vi "ReversedEngineering StateQueuedSettings.vi"(5 "error in (no error)":errorcluster) -> (15 "Cancelled":bool, 19 "error out":errorcluster)   [LabVIEW 2012]
uses:
  <resource>/Framework/Providers/Open_GDS/UML/UMLEditor/UMLEditor_StoredPathes.ctl
  <resource>/Framework/Providers/Open_GDS/UML/ContextHelp/ContextHelp_HelpTexts.ctl
  <resource>/Framework/Providers/Open_GDS/ClassProviders/Common/File/File_StoredPathesActions.ctl
panel:
  in  "Help":bool
  in  "VI-Name":string caption="VI-Name that inserts an array of states-transitions\nin the queued state machine."
  in  "Cancel Button":bool
  in  "OK Button":bool
  in  "Path":path
  # "E.g."
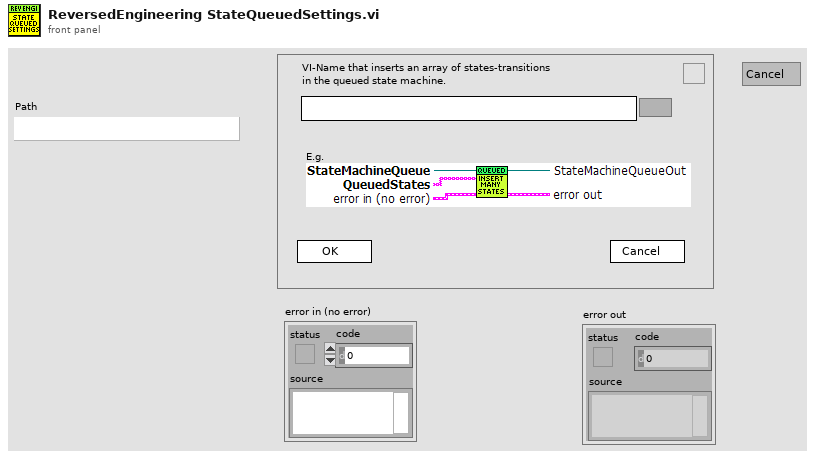
[diagram p1: front panel]
types:
  T1 = typedef "UMLEditor_StoredPathes.ctl" = enum16{"LastSearchPath", "QueuedArrayStateVI", "ClassBasePath", "ViTemplatePath", "ApplicationTemplatePath", "IniFilePath", "WizDir", "RevPlugInPath"}
  T2 = typedef "ContextHelp_HelpTexts.ctl" = enum16{"None(Hide)", "Default", "Help", "Welcome", "GettingStarted", "ClassDiagram_Help", "SequenceDiagram_Help", "UseCaseDiagram_Help", "BSelect", "BClass", "BInterface", "BPackage", "BNote", "BDependency", "BInheritance", "BInterfaceImplementation", "BAssociation", "BAggregation", "BCompAggregation", "BNoteConnector", "BObject", "BActionBar", "BCall", "BSystem", "BActor", "BUseCase", "BGeneralization", "BIncludes", "BExtends", "BUseCaseDiagramAssociation", "ClassRelationshipEdge editDialog_Bent Style", "ClassRelationshipEdge editDialog_RelationType", "ClassRelationshipEdge editDialog_Reverse association", "ClassRelationshipEdge editDialog_Start label", "ClassRelationshipEdge editDialog_Middle label", "ClassRelationshipEdge editDialog_End label", "UMLEditor reversedEngineering_Pathes", "ReversedEngineering StateReverseDialog_Help", "ReversedEngineering StateQueuedSettings_Help", "UMLEditor reversedEngineering_AddTopVIs", "UMLEditor reversedEngineering_AddClasses", "UMLEditor reversedEngineering_AddDirs", "UMLEditor reversedEngineering_Recursively", "UMLEditor reversedEngineering_Remove", "UMLEditor reversedEngineering_ClearList", "UMLEditor reversedEngineering_HideSubAss", "UMLEditor reversedEngineering_CreateTypes", "UMLEditor reversedEngineering_OnlyInheritance", "UMLEditor reversedEngineering_CreateApplication", "UMLEditor reversedEngineering_OK", "UMLEditor reversedEngineering_Cancel", "UMLEditor reversedEngineering_Help", "UMLEditor createWizardScriptFile_ScriptfilePath", "UMLEditor createWizardScriptFile_ClassPath", "UMLEditor createWizardScriptFile_Use", "UMLEditor createWizardScriptFile_PrivateDirName", "UMLEditor createWizardScriptFile_DirAppend", "UMLEditor createWizardScriptFile_Separator Character", "UMLEditor createWizardScriptFile_OK", "UMLEditor createWizardScriptFile_Cancel", "UMLEditor createWizardScriptFile_Help", "ClassNode editDialog_Class Name", "InterfaceNode editDialog_Class Name", "ClassNode editDialog_Attribute", "ClassNode editDialog_Methods", "InterfaceNode editDialog_Methods", "ClassNode editDialog_connection", "InterfaceNode editDialog_connection", "ClassNode editDialog_StereoType", "ClassNode editDialog_ShowAttrib", "ClassNode editDialog_ShowMethods", "ClassNode editDialog_ClassPath", "ClassNode editDialog_AddAttribute", "ClassNode editDialog_AddMethod", "InterfaceNode editDialog_AddMethod", "ClassNode AttributeGuide_AttributeName", "ClassNode AttributeGuide_Array?", "ClassNode AttributeGuide_Data Type", "ClassNode AttributeGuide_RefName", "ClassNode AttributeGuide_Preview", "ClassNode AttributeGuide_OK", "ClassNode AttributeGuide_Cancel", "ClassNode MethodGuide_Visibility", "ClassNode MethodGuide_Method Name", "ClassNode MethodGuide_Preview", "ClassNode MethodGuide_OK", "ClassNode MethodGuide_Cancel", "CallNode EditCallProperties_AllButtons", "ObjectNode EditObjectlProperties_AllButtons", "ActorNode EditActorProperties_AllButtons", "UseCaseRelationshipNode EditUseCaselProperties_AllButtons", "UseCaseNode EditUseCaselProperties_AllButtons", "SystemNode EditSystemProperties_AllButtons", "ReversedEngineering UpdateAttributes_AllButtons", "StateNode editDialog_AllButtons", "StateTransition editDialog_AllButtons", "ArrangeNodes Main_Picture", "ArrangeNodes Main_Zoom", "ArrangeNodes Main_Auto Zoom", "ArrangeNodes Main_shorten", "ArrangeNodes Main_Min Length", "ArrangeNodes Main_Max Length", "ArrangeNodes Main_increase", "ArrangeNodes Main_decrease", "ArrangeNodes Main_Shake", "ArrangeNodes Main", "BState", "BInitialState", "BFinalState", "BStateTransition", "StateDiagram_Help", "StateDiagram_PropertiesAllButtons", "ReversedEngineering StateReverseDialog_ClearStates", "ReversedEngineering StateReverseDialog_UseQueuedStateMachines", "ReversedEngineering StateReverseDialog_QueuedSettings", "ReversedEngineering StateReverseDialog_SearchForVIs", "ReversedEngineering StateReverseDialog_SearchCriteria", "OptionsDialog_ClassBasePath", "OptionsDialog_VIPath", "OptionsDialog_ApplicationPath", "OptionsDialog_WizDir", "OptionsDialog_IniFilePath", "OptionsDialog_DefineColors", "OptionsDialog_Help", "OptionsDialog_CreateTypes", "ClassRelationshipEdge editDialog_SplitWire"}
  T3 = typedef "ContextHelp_ShowType.ctl" = cluster{"Header":string, "Picture":picture, "Text":string}
  T4 = typedef "File_StoredPathesActions.ctl" = enum16{"Get Path", "Set Path", "Delete Path", "Clear All Paths"}
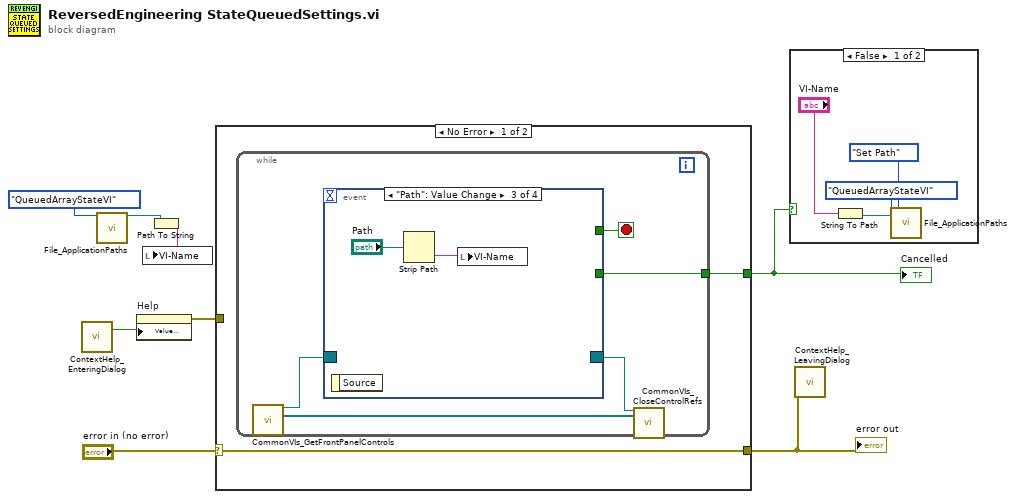
[diagram p0: block diagram]
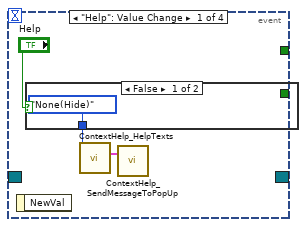
[diagram p3: hidden frame]
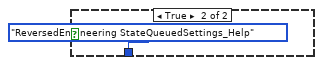
[diagram p4: hidden frame]
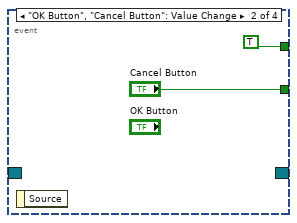
[diagram p5: hidden frame]
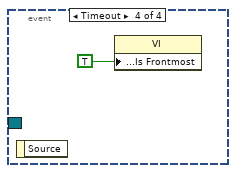
[diagram p6: hidden frame]
diagram:
  n1 = call <resource>:"ContextHelp_EnteringDialog.vi"() -> ("HelpStatus"=w7:bool)  [unwired: 1 in, 18 out]
  n2 = call <resource>:"File_ApplicationPaths.vi"("PathName"=UMLEditor_StoredPathes."QueuedArrayStateVI" ("UMLPathes")) -> ("Path Out"=w2:path)  [unwired: 3 in, 15 out]
  n3 = property on="Help" class="Bool (strict)"("Value (Signaling)"=w7) -> (error out=w6:errorcluster)  [unwired: 2 in, 1 out]
  n4 = Path To String(path=w2) -> (string=w1:string)
  n5 = local write "VI-Name"(w1) -> ()
  n6 = case shown="No Error" "error in (no error)" {
    selector: "error in (no error)" -> [w10 w26]
    tunnel: [w10 w26] -> w5
    tunnel: w6 -> [_ _]
    tunnel: [w9 _] -> w4
    frame No Error {
      n7 = while {
        tunnel: [w11] -> w9
        stop <- w12 stop-if-true
        n8 = call <resource>:"CommonVIs_GetFrontPanelControls.vi"() -> ("Event Registration Refnum"=w14:refnum<event-registration>, "ControlRefs"=w15:refnum<vi>[])  [unwired: 2 in, 16 out]
        n9 = event shown="[2] \"Path\": Value Change" {
          selector: w14 -> [_ _ _ _]
          dyn-events: [_ _ _ _] -> w13
          timeout: _ -> [_ _ _ _]
          tunnel: [_ TRUE _ _] -> w12
          tunnel: [_ "Cancel Button" _ _] -> w11
          event "Help": Value Change {
            n10 = event-data() -> ()  [unwired: 2 out]
            n11 = case shown="False" "Help" {
              tunnel: [ContextHelp_HelpTexts."None(Hide)" ("HelpText") ContextHelp_HelpTexts."ReversedEngineering StateQueuedSettings_Help" ("HelpText")] -> w18
              frame False {
              }
              frame True {
              }
            }
            n12 = call <resource>:"ContextHelp_HelpTexts.vi"("HelpText (enum or string)"=w18) -> ("HelpOut"=w17:T3)  [unwired: 18 out]
            n13 = call <resource>:"ContextHelp_SendMessageToPopUp.vi"("PopUpMessage"=w17) -> ()  [unwired: 2 in, 17 out]
          }
          event "OK Button", "Cancel Button": Value Change {
            n14 = event-data() -> ()  [unwired: 2 out]
          }
          event "Path": Value Change {
            n15 = event-data() -> ()  [unwired: 2 out]
            n16 = Strip Path(path="Path") -> (name=w23:string)  [unwired: 1 out]
            n17 = local write "VI-Name"(w23) -> ()
          }
          event Timeout {
            n18 = event-data() -> ()  [unwired: 2 out]
            n19 = property class="VI"("Front Panel Window:Is Frontmost"=TRUE ("Front Panel Window:Open")) -> ()  [unwired: 2 in, 2 out]
          }
        }
        n20 = call <resource>:"CommonVIs_CloseControlRefs.vi"("Event Registration Refnum"=w13, "ControlRefs"=w15) -> ()  [unwired: 1 in, 17 out]
      }
    }
    frame Error {
    }
  }
  "Cancelled" <- w4
  "error out" <- w5
  n21 = case shown="False" w4 {
    frame False {
      n22 = String To Path(string="VI-Name") -> (path=w28:path)
      n23 = call <resource>:"File_ApplicationPaths.vi"("PathName"=UMLEditor_StoredPathes."QueuedArrayStateVI" ("UMLPathes"), "Path In"=w28, "Method (Get Path)"=File_StoredPathesActions."Set Path") -> ()  [unwired: 1 in, 16 out]
    }
    frame True {
    }
  }
  n24 = call <resource>:"ContextHelp_LeavingDialog.vi"("error in (no error)"=w5) -> ()  [unwired: 19 out]
